vi "Main Programv.vi"() -> ()   [LabVIEW 2018]
panel:
  out "In Water Temp Evaporator 7":dbl[unit]
  out "Evaporator current Water Flow Voltage Level 5":dbl
  out "Evaporator Zero Water Flow Voltage Level 2":dbl
  out "Water Flow Eva":bool
  out "Pre Evaporation Water Flow Detected by sensor":dbl[unit](slide)
  out "Pre Evaporation Water Flow Detected by sensor":dbl[unit]
  out "S1 is greater Than S2\nThat is Wrong":bool
  out "Orifice Air current AIR Flow Voltage Level 4":dbl
  out "Air Flow":bool
  out "Water Flow Pre Eva":bool
  out "T_WD":dbl[unit]
  out "T_WD\nEvaporator Outlet Cold \nWater Temprature":dbl[unit](slide) scale=15.0..70.0
  out "Temprature Of Output Air Centigrade Degree":dbl[unit](slide) scale=15.0..70.0
  out "LMTD":dbl[unit](knob) scale=0.0..5.0
  out "LMTD":dbl[unit]
  out "Out Water Temp of Pre Evaporator 2":dbl[unit]
  out "AIR temp Evaporator In 3":dbl[unit]
  out "AIR temp Evaporator Out 4":dbl[unit]
  out "In Water Temp Evaporator 6":dbl[unit]
  out "Pre Evaporator current Water Flow Voltage Level 4":dbl
  out "Pre Evaporator Zero Water Flow Voltage Level 2":dbl
  out "In Water Temp Pre Evaporator 2":dbl[unit]
  out "AIR temp Evaporator Out 3":dbl[unit]
  out "AIR temp Evaporator In 2":dbl[unit]
  out "Humidity of Evaporator Out 3":dbl
  out "Orifice Air Ziro AIR Flow Voltage Level 2":dbl
  out "Orifice Air current AIR Flow Voltage Level 3":dbl
  out "Humidity of Evaporator In 3":dbl
  out "In Water Temp Evaporator 2":dbl[unit]
  out "Out Water Temp Evaporator 3":dbl[unit]
  out "Evaporation Water Flow Detected by sensor":dbl[unit]
  out "Evaporation Water Flow Detected by sensor":dbl[unit](slide)
  out "Temprature Of Input Air\nCentigrade Degree":dbl[unit](slide) scale=15.0..70.0
  out "Humidity of Input Air 2":dbl(knob) scale=30.0..100.0
  out "T_WU":dbl[unit]
  out "T_WU\nEvaporator Inlet Hot \nWater Temprature":dbl[unit](slide) scale=15.0..70.0
  out "MFRHA\nMass Flow Rate of Humid Air \nof Input(Kg/s)":dbl[unit]
  out "Added Vapor (kg/s)":dbl[unit]
  out "Total Transferd Energy of Air":dbl[unit]
  out "Mass FLow Rate of \nOutput Expose Saline Water":dbl[unit]
  out "Mass FLow Rate of \nInput Expose Saline Water":dbl[unit]
  out "Total Enthalphy of \nOut Put Exposed Saline Water":dbl[unit]
  out "Total Enthalphy of In Put Exposed Saline Water":dbl[unit]
  out "Total Transfered Energy from Exposed Saline Water 2":dbl[unit]
  out "Mass FLow Rate of \nInput Expose Saline Water":dbl[unit](slide)
  out "Total Transferd Energy of Air":dbl[unit](knob)
  out "Mass Flow Rate of Coil Water":dbl[unit]
  out "Mass Flow Rate of Coil Water":dbl[unit](slide)
  out "Tceg":dbl[unit]
  out "Humidity of Input Air":dbl
  in  "Gas Presure":dbl[unit]=80000.0 min=80000.0 max=120000.0
  out "Humidity of Evaporator Out\nRH Heat Exchanger Quality":dbl
  out "Humidity of Evaporator Out\nRH Heat Exchanger Quality":dbl(knob) scale=30.0..100.0
  out "temp Evaporator In 3":dbl[unit]
  out "Evaporator Out 4":dbl[unit]
  out "temp Evaporator In 2":dbl[unit]
  out "Evaporator Out 3":dbl[unit]
  out "Pre Evaporator Out 3":dbl[unit]
  out "Evaporator current Water Flow Voltage Level 4":dbl
  out "Series 4":dbl[unit]
  out "Evaporator In":dbl[unit]
  out "Evaporator current Water Flow Voltage Level 3":dbl
  out "Pre Evaporator current Water Flow Voltage Level 3":dbl
  out "In Water Temp Evaporator 3":dbl[unit]
  out "In Water Temp Evaporator 4":dbl[unit]
  out "Humidity of Evaporator In 4":dbl
  out "In Water Temp Evaporator 5":dbl[unit]
  out "AIR temp Evaporator Out 2":dbl[unit]
  out "Out Water Temp Evaporator 2":dbl[unit]
  out "Out Air temp Evaporator":dbl[unit]
  in  "stop":bool
  in  "Calibration":bool
  in  "Run Program":bool
  out "Humidity of Evaporator In 2":dbl
  out "Humidity of Evaporator Out 2":dbl
  out "temp Evaporator In":dbl[unit]
  out "temp Evaporator Out 2":dbl[unit]
  out "broken air humidity sensor":dbl
  out "Humidity of Evaporator In":dbl
  out "Humidity of Evaporator Out":dbl
  out "broken air temp sensor":dbl[unit]
  out "AIR temp Evaporator In":dbl[unit]
  out "AIR temp Evaporator Out":dbl[unit]
  out "Orifice Air current AIR Flow Voltage Level 2":dbl
  out "Pre Evaporator current Water Flow Voltage Level 2":dbl
  out "Evaporator current Water Flow Voltage Level 2":dbl
  out "Orifice Air current AIR Flow Voltage Level":dbl
  out "Pre Evaporator current Water Flow Voltage Level":dbl
  out "Evaporator current Water Flow Voltage Level":dbl
  out "Orifice Air Ziro AIR Flow Voltage Level 3":dbl
  out "Pre Evaporator Zero Water Flow Voltage Level 3":dbl
  out "Evaporator Zero Water Flow Voltage Level4":dbl
  out "Evaporator Zero Water Flow Voltage Level":dbl
  out "Orifice Air Ziro AIR Flow Voltage Level":dbl
  out "Pre Evaporator Zero Water Flow Voltage Level":dbl
  out "Series 3":dbl[unit]
  out "Evaporator Out 2":dbl[unit]
  out "Pre Evaporator In":dbl[unit]
  out "Series 2":dbl[unit]
  out "Out Water Temp Evaporator":dbl[unit]
  out "In Water Temp Pre Evaporator":dbl[unit]
  out "Pre Evaporator Out 2":dbl[unit]
  out "Evaporator In 2":dbl[unit]
  out "In Water Temp Evaporator":dbl[unit]
  out "Out Water Temp of Pre Evaporator":dbl[unit]
  out "Run Trip":i32
  out "E1":i32
  out "E2":i32
  out "E3":i32
  out "E4":i32
  out "EEP":string
  out "eep":bool
  out "M1":i32
  out "M2":i32
  out "M3":i32
  out "M4":i32
  out "MPXV7002":string
  out "mpxv":bool
  out "S1":i32
  out "S2":i32
  out "S3":i32
  out "S4":i32
  out "SHT11":string
  out "sht":bool
  out "D1":i32
  out "D2":i32
  out "D3":i32
  out "D4":i32
  out "ds18b20":string
  out "ds":bool
  out "PortName":string
  out "GetPortNames":string[](array[string])
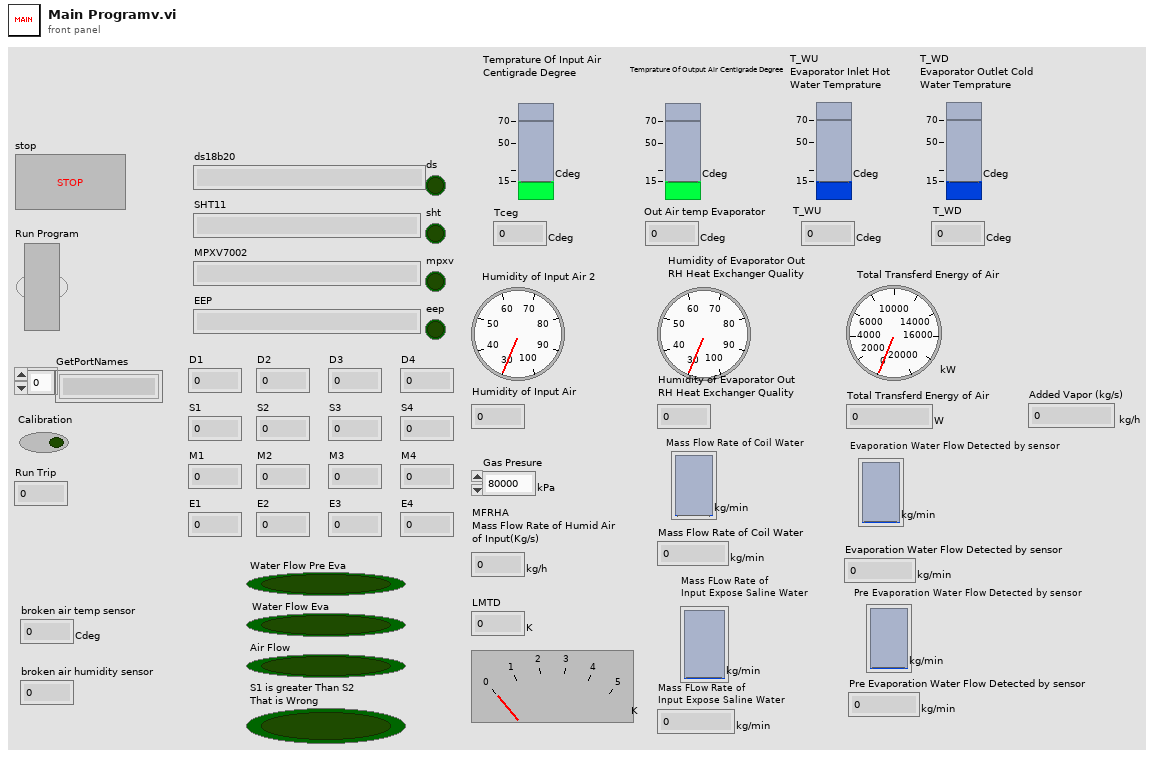
[diagram p1: front panel]
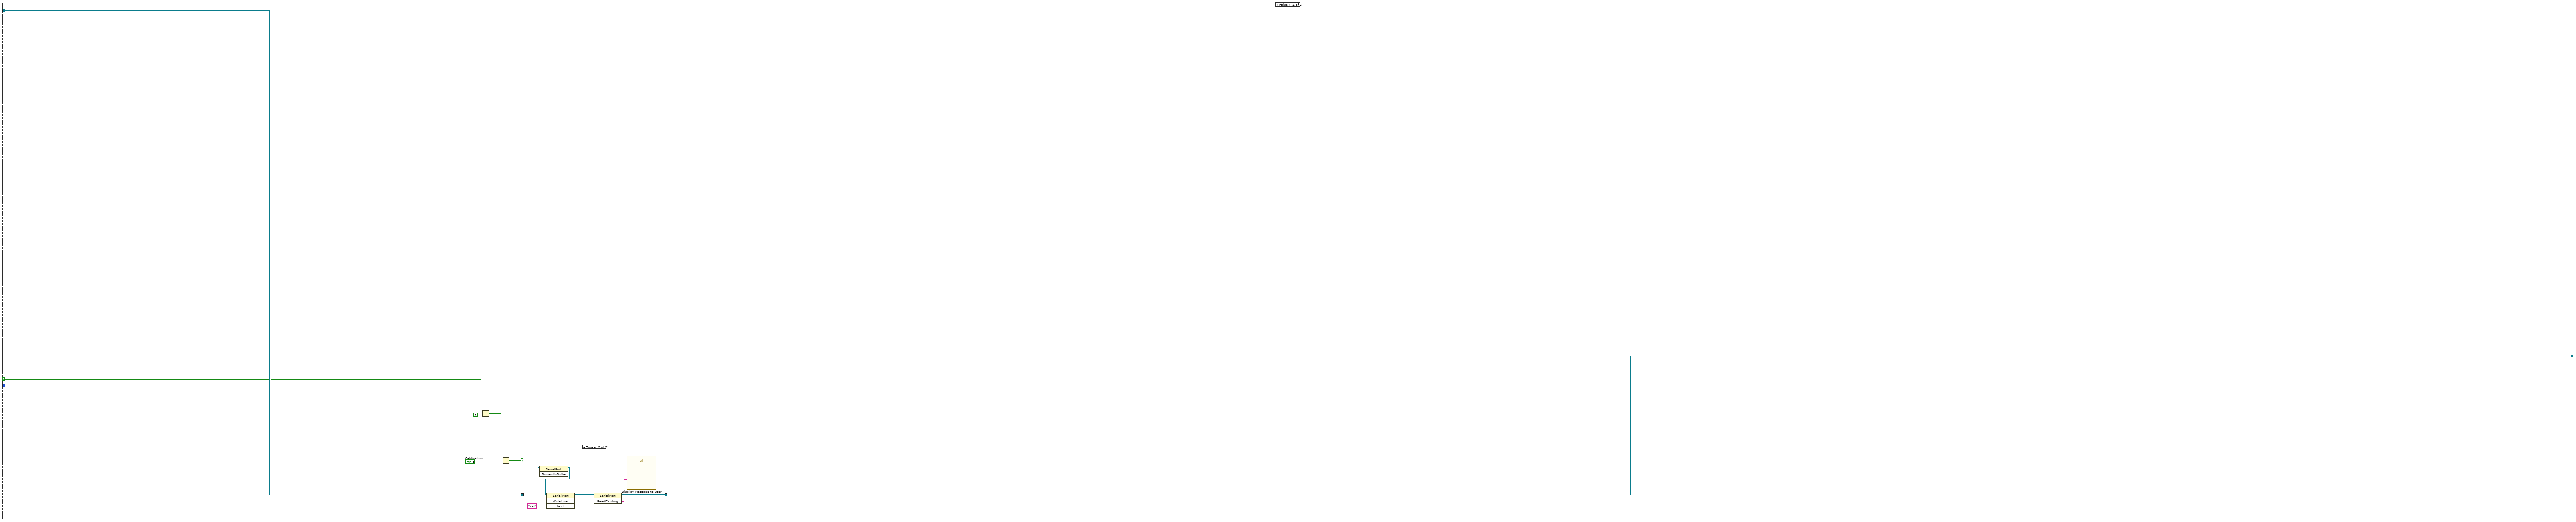
[diagram p2: hidden frame]
diagram:
  w7 = 1 items=["None", "One", "Two", "OnePointFive"] ("StopBits")
  w6 = 0 items=["None", "Odd", "Even", "Mark", "Space"] ("Parity")
  n1 = constructor class="SerialPort"() -> (reference out=w12:refnum<k24>, error out=w13:errorcluster)  [unwired: 3 in, 1 out]
  n2 = local read "GetPortNames"() -> (w16:string[])
  n3 = invoke class="SerialPort" method="GetPortNames"(reference=w12, error in=w13) -> (reference out=w14:refnum<k24>, "GetPortNames"=→"GetPortNames":string[])  [unwired: 1 in, 1 out]
  n4 = Index Array(array=w16, index=0) -> (element=→"PortName":string)
  n5 = local read "PortName"() -> (w11:string)
  n6 = property class="SerialPort"(reference=w14, "PortName"=w11) -> (reference out=w3:refnum<k24>)  [unwired: 1 in, 1 out]
  n7 = property class="SerialPort"(reference=w3, "DataBits"=8) -> ()  [unwired: 1 in, 2 out]
  n8 = property class="SerialPort"(reference=w3, "BaudRate"=57600) -> ()  [unwired: 1 in, 2 out]
  n9 = property class="SerialPort"(reference=w3, "StopBits"=w7) -> ()  [unwired: 1 in, 2 out]
  n10 = invoke class="SerialPort" method="Open"(reference=w3) -> (reference out=w9:refnum<k24>)  [unwired: 2 in, 2 out]
  n11 = property class="SerialPort"(reference=w3, "Parity"=w6) -> ()  [unwired: 1 in, 2 out]
  n12 = local write "Run Trip"(0 ("Run Trip")) -> ()
  n13 = property class="SerialPort" props=["IsOpen"](reference=w9) -> (reference out=w4:refnum<k24>)  [unwired: 1 in, 2 out]
  n14 = while {
    tunnel: w4 -> [w26]
    tunnel: [w25] -> w2
    i -> [w21]
    stop <- "stop" stop-if-true
    n15 = local write "Water Flow Pre Eva"(FALSE ("Water Flow Pre Eva")) -> ()
    n16 = local write "Water Flow Eva"(FALSE ("Water Flow Eva")) -> ()
    n17 = local write "Air Flow"(FALSE ("Air Flow")) -> ()
    n18 = case shown="True" "Run Program" {
      selector: "Run Program" -> [w32 _]
      tunnel: w26 -> [w33 w44]
      tunnel: [w27 w43] -> w25
      tunnel: w21 -> [_ w41]
      frame False {
        n19 = Equal?(x=w32, y=FALSE) -> (x = y?=w30:bool)
        n20 = Equal?(x=w30, y="Calibration") -> (x = y?=w28:bool)
        n21 = case shown="True" w28 {
          tunnel: w33 -> [w34 w36]
          tunnel: [w34 w39] -> w27
          frame False {
          }
          frame True {
            n22 = invoke class="SerialPort" method="DiscardInBuffer"(reference=w36) -> (reference out=w35:refnum<k24>)  [unwired: 2 in, 2 out]
            n23 = invoke class="SerialPort" method="WriteLine"(reference=w35, "text"="cal" ("write buffer")) -> (reference out=w40:refnum<k24>)  [unwired: 2 in, 3 out]
            n24 = invoke class="SerialPort" method="ReadExisting"(reference=w40) -> (reference out=w39:refnum<k24>, "ReadExisting"=w37:string)  [unwired: 2 in, 1 out]
            n25 = call "Display Message to User"("Message"=w37) -> ()  [unwired: 9 in, 2 out]
          }
        }
      }
      frame True {
        n26 = flat-sequence {
          tunnel: [w64] -> w62
          tunnel: w44 -> [w63]
          tunnel: w62 -> [w70]
          tunnel: [w69] -> w61
          tunnel: w61 -> [w79]
          tunnel: [w79] -> w60
          tunnel: w41 -> [w71]
          tunnel: w60 -> [w122]
          tunnel: [w119] -> w59
          tunnel: w59 -> [w125]
          tunnel: [w124] -> w58
          tunnel: w58 -> [w134]
          tunnel: [w134] -> w57
          tunnel: w57 -> [w176]
          tunnel: [w175] -> w56
          tunnel: w56 -> [w182]
          tunnel: [w180] -> w55
          tunnel: w55 -> [w190]
          tunnel: [w190] -> w54
          tunnel: w54 -> [w219]
          tunnel: [w216] -> w53
          tunnel: w53 -> [w222]
          tunnel: [w221] -> w52
          tunnel: w52 -> [w231]
          tunnel: [w231] -> w51
          tunnel: [w257] -> w50
          tunnel: w51 -> [w257]
          tunnel: w50 -> [w263]
          tunnel: [w263] -> w49
          tunnel: w49 -> [w265]
          tunnel: [w264] -> w48
          tunnel: [w293] -> w43
          tunnel: w48 -> [w293]
          frame #0 {
            n27 = Wait (ms)(milliseconds to wait=u32 2000) -> ()  [unwired: 1 out]
            n28 = invoke class="SerialPort" method="WriteLine"(reference=w63, "text"="ds18b20") -> (reference out=w64:refnum<k24>)  [unwired: 2 in, 3 out]
          }
          frame #1 {
            n29 = invoke class="SerialPort" method="ReadExisting"(reference=w70) -> (reference out=w69:refnum<k24>, "ReadExisting"=→"ds18b20":string)  [unwired: 2 in, 1 out]
            "ds" <- TRUE ("DS")
          }
          frame #2 {
            n30 = local read "ds18b20"() -> (w73:string)
            n31 = call "DVFS.vi"("Start string"="*", "string"=w73, "end string"="#") -> ("Output"=w72:i32[])  [unwired: 3 in, 2 out]
            n32 = Index Array(array=w72, index=0) -> (element=w75:i32)
            n33 = Not Equal To 0?(x=w75) -> (x != 0?=w74:bool)
            n34 = case shown="True" w74 {
              tunnel: w72 -> [_ w118]
              frame False {
              }
              frame True {
                n35 = Index Array(array=w118, index #1=0 ("index"), index #2=1 ("index"), index #3=2 ("index"), index #4=3 ("index"), index #5=4 ("index"), index #6=5 ("index"), index #7=6 ("index"), index #8=7 ("index")) -> (element #1=w86:i32, element #2=w85:i32, element #3=w84:i32, element #4=w83:i32, element #5=w82:i32)  [unwired: 3 out]
                "D1" <- w86
                "D2" <- w85
                "D3" <- w84
                "D4" <- w83
                n36 = To Double Precision Float(number=w86) -> (double precision float=w109:dbl)
                n37 = To Double Precision Float(number=w85) -> (double precision float=w104:dbl)
                n38 = To Double Precision Float(number=w84) -> (double precision float=w101:dbl)
                n39 = To Double Precision Float(number=w83) -> (double precision float=w99:dbl)
                n40 = To Double Precision Float(number=w82) -> (double precision float=w94:dbl)
                n41 = Divide(x=w109, y=100.0) -> (x/y=w107:dbl)
                n42 = Divide(x=w104, y=100.0) -> (x/y=w81:dbl)
                n43 = Divide(x=w101, y=100.0) -> (x/y=w80:dbl)
                n44 = Divide(x=w99, y=100.0) -> (x/y=w95:dbl)
                n45 = Divide(x=w94, y=100.0) -> (x/y=w91:dbl)
                n46 = node(w107) -> (→"Out Water Temp of Pre Evaporator":dbl[unit])
                n47 = node(w81) -> (→"In Water Temp Evaporator":dbl[unit])
                n48 = node(w80) -> (→"In Water Temp Pre Evaporator":dbl[unit])
                n49 = node(w95) -> (→"Out Water Temp Evaporator":dbl[unit])
                n50 = node(w91) -> (→"Series 2":dbl[unit])
                n51 = local read "Out Water Temp Evaporator"() -> (→"Evaporator Out 2":dbl[unit])
                n52 = local read "In Water Temp Evaporator"() -> (→"Evaporator In 2":dbl[unit])
                n53 = local read "In Water Temp Pre Evaporator"() -> (→"Pre Evaporator In":dbl[unit])
                n54 = local read "Out Water Temp of Pre Evaporator"() -> (→"Pre Evaporator Out 2":dbl[unit])
                n55 = local read "Series 2"() -> (→"Series 3":dbl[unit])
              }
            }
            "Run Trip" <- w71
          }
          frame #3 {
            n56 = Wait (ms)(milliseconds to wait=u32 4000) -> ()  [unwired: 1 out]
            n57 = invoke class="SerialPort" method="WriteLine"(reference=w122, "text"="sht11" ("write buffer")) -> (reference out=w119:refnum<k24>)  [unwired: 2 in, 3 out]
          }
          frame #4 {
            n58 = invoke class="SerialPort" method="ReadExisting"(reference=w125) -> (reference out=w124:refnum<k24>, "ReadExisting"=→"SHT11":string)  [unwired: 2 in, 1 out]
            "sht" <- TRUE ("SHT")
          }
          frame #5 {
            n59 = local read "SHT11"() -> (w128:string)
            n60 = call "DVFS.vi"("Start string"="*", "string"=w128, "end string"="/") -> ("Output"=w127:i32[])  [unwired: 3 in, 2 out]
            n61 = Index Array(array=w127, index=0) -> (element=w130:i32)
            n62 = Not Equal To 0?(x=w130) -> (x != 0?=w129:bool)
            n63 = case shown="True" w129 {
              tunnel: w127 -> [_ w174]
              frame False {
              }
              frame True {
                n64 = Index Array(array=w174, index #1=0 ("index"), index #2=1 ("index"), index #3=2 ("index"), index #4=3 ("index"), index #5=4 ("index"), index #6=5 ("index"), index #7=6 ("index"), index #8=7 ("index")) -> (element #1=w144:i32, element #2=w143:i32, element #3=w142:i32, element #4=w141:i32, element #5=w140:i32, element #6=w139:i32)  [unwired: 2 out]
                "S1" <- w144
                "S2" <- w143
                "S3" <- w142
                "S4" <- w141
                n65 = To Double Precision Float(number=w144) -> (double precision float=w165:dbl)
                n66 = To Double Precision Float(number=w143) -> (double precision float=w155:dbl)
                n67 = To Double Precision Float(number=w142) -> (double precision float=w163:dbl)
                n68 = To Double Precision Float(number=w141) -> (double precision float=w153:dbl)
                n69 = To Double Precision Float(number=w140) -> (double precision float=w161:dbl)
                n70 = To Double Precision Float(number=w139) -> (double precision float=w150:dbl)
                n71 = Divide(x=w165, y=100.0) -> (x/y=w137:dbl)
                n72 = Divide(x=w155, y=100.0) -> (x/y=→"Humidity of Evaporator Out":dbl)
                n73 = Divide(x=w163, y=100.0) -> (x/y=w157:dbl)
                n74 = Divide(x=w153, y=100.0) -> (x/y=→"Humidity of Evaporator In":dbl)
                n75 = Divide(x=w161, y=100.0) -> (x/y=w136:dbl)
                n76 = Divide(x=w150, y=100.0) -> (x/y=→"broken air humidity sensor":dbl)
                n77 = node(w157) -> (→"AIR temp Evaporator In":dbl[unit])
                n78 = node(w137) -> (→"AIR temp Evaporator Out":dbl[unit])
                n79 = node(w136) -> (→"broken air temp sensor":dbl[unit])
                n80 = local read "AIR temp Evaporator Out"() -> (→"temp Evaporator Out 2":dbl[unit])
                n81 = local read "Humidity of Evaporator Out"() -> (→"Humidity of Evaporator Out 2":dbl)
                n82 = local read "AIR temp Evaporator In"() -> (→"temp Evaporator In":dbl[unit])
                n83 = local read "Humidity of Evaporator In"() -> (→"Humidity of Evaporator In 2":dbl)
              }
            }
          }
          frame #6 {
            n84 = Wait (ms)(milliseconds to wait=u32 5000) -> ()  [unwired: 1 out]
            n85 = invoke class="SerialPort" method="WriteLine"(reference=w176, "text"="mpxv7002" ("write buffer")) -> (reference out=w175:refnum<k24>)  [unwired: 2 in, 3 out]
          }
          frame #7 {
            n86 = invoke class="SerialPort" method="ReadExisting"(reference=w182) -> (reference out=w180:refnum<k24>, "ReadExisting"=→"MPXV7002":string)  [unwired: 2 in, 1 out]
            "mpxv" <- TRUE ("MPXV")
          }
          frame #8 {
            n87 = local read "MPXV7002"() -> (w184:string)
            n88 = call "DVFS.vi"("Start string"="*", "string"=w184, "end string"="+") -> ("Output"=w183:i32[])  [unwired: 3 in, 2 out]
            n89 = Index Array(array=w183, index=0) -> (element=w186:i32)
            n90 = Not Equal To 0?(x=w186) -> (x != 0?=w185:bool)
            n91 = case shown="True" w185 {
              tunnel: w183 -> [_ w215]
              frame False {
              }
              frame True {
                n92 = Index Array(array=w215, index #1=0 ("index"), index #2=1 ("index"), index #3=2 ("index"), index #4=3 ("index"), index #5=4 ("index"), index #6=5 ("index"), index #7=6 ("index"), index #8=7 ("index")) -> (element #1=w193:i32, element #2=w192:i32, element #3=w191:i32, element #4=→"M4":i32)  [unwired: 4 out]
                "M1" <- w193
                "M2" <- w192
                "M3" <- w191
                n93 = local read "Orifice Air current AIR Flow Voltage Level"() -> (→"Orifice Air current AIR Flow Voltage Level 2":dbl)
                n94 = local read "Evaporator current Water Flow Voltage Level"() -> (→"Evaporator current Water Flow Voltage Level 2":dbl)
                n95 = local read "Pre Evaporator current Water Flow Voltage Level"() -> (→"Pre Evaporator current Water Flow Voltage Level 2":dbl)
                n96 = To Double Precision Float(number=w193) -> (double precision float=w205:dbl)
                n97 = To Double Precision Float(number=w192) -> (double precision float=w203:dbl)
                n98 = To Double Precision Float(number=w191) -> (double precision float=w201:dbl)
                n99 = Divide(x=w205, y=100.0) -> (x/y=→"Evaporator current Water Flow Voltage Level":dbl)
                n100 = Divide(x=w203, y=100.0) -> (x/y=→"Pre Evaporator current Water Flow Voltage Level":dbl)
                n101 = Divide(x=w201, y=100.0) -> (x/y=→"Orifice Air current AIR Flow Voltage Level":dbl)
              }
            }
          }
          frame #9 {
            n102 = invoke class="SerialPort" method="WriteLine"(reference=w219, "text"="EEP" ("write buffer")) -> (reference out=w216:refnum<k24>)  [unwired: 2 in, 3 out]
            n103 = Wait (ms)(milliseconds to wait=u32 1000) -> ()  [unwired: 1 out]
          }
          frame #10 {
            n104 = invoke class="SerialPort" method="ReadExisting"(reference=w222) -> (reference out=w221:refnum<k24>, "ReadExisting"=→"EEP":string)  [unwired: 2 in, 1 out]
            "eep" <- TRUE ("EEP")
          }
          frame #11 {
            n105 = local read "EEP"() -> (w225:string)
            n106 = call "DVFS.vi"("Start string"="*", "string"=w225, "end string"="-") -> ("Output"=w224:i32[])  [unwired: 3 in, 2 out]
            n107 = Index Array(array=w224, index=0) -> (element=w227:i32)
            n108 = Not Equal To 0?(x=w227) -> (x != 0?=w226:bool)
            n109 = case shown="True" w226 {
              tunnel: w224 -> [_ w256]
              frame False {
              }
              frame True {
                n110 = Index Array(array=w256, index #1=0 ("index"), index #2=1 ("index"), index #3=2 ("index"), index #4=3 ("index"), index #5=4 ("index"), index #6=5 ("index"), index #7=6 ("index"), index #8=7 ("index")) -> (element #1=w234:i32, element #2=w232:i32, element #3=w233:i32, element #4=→"E4":i32)  [unwired: 4 out]
                "E1" <- w234
                "E2" <- w232
                "E3" <- w233
                n111 = local read "Evaporator Zero Water Flow Voltage Level"() -> (→"Evaporator Zero Water Flow Voltage Level4":dbl)
                n112 = local read "Pre Evaporator Zero Water Flow Voltage Level"() -> (→"Pre Evaporator Zero Water Flow Voltage Level 3":dbl)
                n113 = local read "Orifice Air Ziro AIR Flow Voltage Level"() -> (→"Orifice Air Ziro AIR Flow Voltage Level 3":dbl)
                n114 = To Double Precision Float(number=w234) -> (double precision float=w246:dbl)
                n115 = To Double Precision Float(number=w232) -> (double precision float=w244:dbl)
                n116 = To Double Precision Float(number=w233) -> (double precision float=w242:dbl)
                n117 = Divide(x=w246, y=100.0) -> (x/y=→"Evaporator Zero Water Flow Voltage Level":dbl)
                n118 = Divide(x=w244, y=100.0) -> (x/y=→"Pre Evaporator Zero Water Flow Voltage Level":dbl)
                n119 = Divide(x=w242, y=100.0) -> (x/y=→"Orifice Air Ziro AIR Flow Voltage Level":dbl)
              }
            }
          }
          frame #12 {
            n120 = Wait (ms)(milliseconds to wait=u32 1000) -> ()  [unwired: 1 out]
          }
          frame #13 {
            n121 = local write "mpxv"(FALSE ("mpxv")) -> ()
            n122 = local write "ds"(FALSE ("eep")) -> ()
            n123 = local write "eep"(FALSE ("DS")) -> ()
            n124 = local write "sht"(FALSE ("sht")) -> ()
          }
          frame #14 {
            n125 = invoke class="SerialPort" method="DiscardInBuffer"(reference=w265) -> (reference out=w264:refnum<k24>)  [unwired: 2 in, 2 out]
            n126 = invoke class="SerialPort" method="DiscardOutBuffer"(reference=w265) -> ()  [unwired: 2 in, 3 out]
          }
          frame #15 {
            w280 = 0.004 ("Salinity of Output Exposed\n Saline Water")
            w281 = 0.0035 ("Salinity of Input Exposed \nSaline Water")
            w315 = dbl[unit] 0.12  # Air Pipe Diameter (mm)
            w316 = dbl[unit] 0.05  # Air Orifice Diameter
            w288 = dbl[unit] 0.0075  # Water Orifice Diameter (mm) In Pre Evaporation
            n127 = local read "Humidity of Evaporator Out"() -> (w325:dbl)
            "Humidity of Evaporator Out\nRH Heat Exchanger Quality" <- w325
            "Humidity of Evaporator Out\nRH Heat Exchanger Quality" <- w325
            n128 = local read "AIR temp Evaporator Out"() -> (w292:dbl[unit])
            "Out Air temp Evaporator" <- w292
            "Temprature Of Output Air Centigrade Degree" <- w292
            n129 = local read "AIR temp Evaporator In"() -> (w319:dbl[unit])
            "Temprature Of Input Air\nCentigrade Degree" <- w319
            "Tceg" <- w319
            n130 = local read "Orifice Air current AIR Flow Voltage Level"() -> (w287:dbl)
            n131 = local read "Orifice Air Ziro AIR Flow Voltage Level"() -> (w300:dbl)
            n132 = local read "Humidity of Evaporator In"() -> (w320:dbl)
            n133 = local read "In Water Temp Evaporator"() -> (w303:dbl[unit])
            "T_WU" <- w303
            "T_WU\nEvaporator Inlet Hot \nWater Temprature" <- w303
            n134 = local read "Out Water Temp Evaporator"() -> (w323:dbl[unit])
            n135 = local read "Humidity of Evaporator In"() -> (w302:dbl)
            "Humidity of Input Air 2" <- w302
            "Humidity of Input Air" <- w302
            n136 = Subtract(x=w287, y=w300) -> (x-y=w301:dbl)
            n137 = Multiply(x=w301, y=dbl[unit] 4.88) -> (x*y=w317:dbl[unit])
            n138 = call "Orifice Flow Calculation For Air Iso5167.vi"("RH"=w320, "Orifice Diameter"=w316, "Gas Temperature"=w319, "P1\n(Presure After Fan &\n before Orifice)"="Gas Presure", "Pipe Diameter (mm)"=w315, "Delta P\n(Presure Made By Orifice)"=w317) -> ("Mass Flow (Orifice) (Kg/h)"=w304:dbl[unit], "Air Flow"=→"Air Flow":bool)  [unwired: 1 out]
            "MFRHA\nMass Flow Rate of Humid Air \nof Input(Kg/s)" <- w304
            n139 = call "SEPW Specific Enthalpy of Pure Water (KJ to Kg).vi"("Tceg"=w303) -> ("SEPW"=w308:dbl[unit])
            n140 = call "SEPW Specific Enthalpy of Pure Water (KJ to Kg).vi"("Tceg"=w323) -> ("SEPW"=w307:dbl[unit])
            n141 = call "SESW Specific Enthalpy of Saline Water (J to Kg).vi"("Salinity"=w281, "Sailne Water Temprature"=w303) -> ("SESW"=w321:dbl[unit])
            n142 = call "SESW Specific Enthalpy of Saline Water (J to Kg).vi"("Salinity"=w280, "Sailne Water Temprature"=w323) -> ("SESW"=w322:dbl[unit])
            n143 = call "Humid Air Total Transfered Energy Calculator & OutPut Tempratures.vi"("MFRHA\nMass Flow Rate of Humid Air (Kg/s)"=w304, "Gas Presure"="Gas Presure", "T_AU"=w292, "Tceg"=w319, "RH Heat Exchanger Quality"=w325, "RH"=w302) -> ("Mass Flow Rate of Humid Air of Out Put"=w313:dbl[unit], "ToTal Transferd Energy of Air"=w309:dbl[unit])
            "Total Transferd Energy of Air" <- w309
            "Total Transferd Energy of Air" <- w309
            n144 = local read "In Water Temp Evaporator"() -> (w286:dbl[unit])
            n145 = local read "AIR temp Evaporator Out"() -> (w284:dbl[unit])
            n146 = local read "AIR temp Evaporator In"() -> (w283:dbl[unit])
            n147 = local read "Out Water Temp Evaporator"() -> (w285:dbl[unit])
            "T_WD\nEvaporator Outlet Cold \nWater Temprature" <- w285
            "T_WD" <- w285
            n148 = local read "Evaporator current Water Flow Voltage Level"() -> (w269:dbl)
            n149 = local read "Evaporator Zero Water Flow Voltage Level"() -> (w270:dbl)
            n150 = local read "Pre Evaporator current Water Flow Voltage Level"() -> (w296:dbl)
            n151 = local read "Pre Evaporator Zero Water Flow Voltage Level"() -> (w295:dbl)
            n152 = local read "In Water Temp Evaporator"() -> (w324:dbl[unit])
            n153 = Subtract "Transfered Entalpy from Pure Water"(x=w308, y=w307) -> (x-y=w266:dbl[unit])
            n154 = local read "In Water Temp Evaporator"() -> (w268:dbl[unit])
            n155 = call "LMTD.vi"("Air Down/In Temp"=w283, "Air  UP/Out Temp"=w284, "Water Down/out Temp"=w285, "Water Up/In Temp"=w286) -> ("LMTD"=→"LMTD" →"LMTD":dbl[unit])
            n156 = Subtract(x=w313, y=w304) -> (x-y=w278:dbl[unit])
            "Added Vapor (kg/s)" <- w278
            n157 = call "Salinity Relations.vi"("Adde Vapor"=w278, "S2 / Salinity of Output Exposed Saline Water"=w280, "S1 / Salinity of Input Exposed Saline Water"=w281) -> ("S1 is greater Than S2\nThat is Wrong"=→"S1 is greater Than S2\nThat is Wrong":bool, "Output Exposed Saline Water"=w277:dbl[unit], "Input Exposed Saline Water"=w279:dbl[unit])
            "Mass FLow Rate of \nOutput Expose Saline Water" <- w277
            "Mass FLow Rate of \nInput Expose Saline Water" <- w279
            "Mass FLow Rate of \nInput Expose Saline Water" <- w279
            n158 = Multiply(x=w322, y=w277) -> (x*y=w311:dbl[unit])
            "Total Enthalphy of \nOut Put Exposed Saline Water" <- w311
            n159 = Multiply(x=w321, y=w279) -> (x*y=w312:dbl[unit])
            "Total Enthalphy of In Put Exposed Saline Water" <- w312
            n160 = Subtract "Total Transfered Energy \nfrom Exposed Saline Water"(x=w312, y=w311) -> (x-y=w310:dbl[unit])
            "Total Transfered Energy from Exposed Saline Water 2" <- w310
            n161 = Subtract(x=w269, y=w270) -> (x-y=w273:dbl)
            n162 = Subtract(x=w296, y=w295) -> (x-y=w297:dbl)
            n163 = Subtract(x=w309, y=w310) -> (x-y=w306:dbl[unit])
            n164 = Multiply(x=w273, y=dbl[unit] 4.88) -> (x*y=w272:dbl[unit])
            n165 = Multiply(x=w297, y=dbl[unit] 4.88) -> (x*y=w294:dbl[unit])
            n166 = Divide(x=w306, y=w266) -> (x/y=→"Mass Flow Rate of Coil Water" →"Mass Flow Rate of Coil Water":dbl[unit])
            n167 = call "Orifice Flow Calculator of Water In (((Pre))) Evaporation ASME.vi"("Water Temperature"=w268, "Delta P\n(Presure Made By Orifice)"=w272, "Orifice Diameter"=dbl[unit] 0.01) -> ("Water Flow Pre Eva"=→"Water Flow Eva":bool, "Mass Flow (Orifice) (Kg/min)"=→"Pre Evaporation Water Flow Detected by sensor" →"Pre Evaporation Water Flow Detected by sensor":dbl[unit])  [unwired: 1 in, 1 out]
            n168 = call "Orifice Flow Calculator of Water In (((Pre))) Evaporation ASME.vi"("Water Temperature"=w324, "Delta P\n(Presure Made By Orifice)"=w294, "Orifice Diameter"=w288) -> ("Water Flow Pre Eva"=→"Water Flow Pre Eva":bool, "Mass Flow (Orifice) (Kg/min)"=→"Evaporation Water Flow Detected by sensor" →"Evaporation Water Flow Detected by sensor":dbl[unit])  [unwired: 1 in, 1 out]
            n169 = Wait (ms)(milliseconds to wait=u32 1000) -> ()  [unwired: 1 out]
          }
        }
        n170 = local write "ds"(FALSE ("DS")) -> ()
        n171 = local write "sht"(FALSE ("sht")) -> ()
        n172 = local write "mpxv"(FALSE ("mpxv")) -> ()
        n173 = local write "eep"(FALSE ("eep")) -> ()
      }
    }
    n174 = Wait (ms)(milliseconds to wait=u32 200) -> ()  [unwired: 1 out]
  }
  n175 = invoke class="SerialPort" method="Close"(reference=w2) -> ()  [unwired: 2 in, 3 out]
